vi "New Experiment.vi"(3 "error in (no error)":errorcluster, 4 "Experiment in":T1, 5 "Database.lvlib:Data Store.lvclass":refnum<class "Data Store.lvclass">) -> (0 "error out":errorcluster, 1 "Experiment out":T1, 2 "Database.lvlib:Data Store.lvclass 2":refnum<class "Data Store.lvclass">)   [LabVIEW 2012, in "Database.lvlib" / "Data Store.lvclass"]
uses:
  Data Store.lvclass
  Experiment.ctl
  <vilib>/addons/database/Auxilliary.llb/DB Tools Isolation Level.ctl
  <vilib>/addons/database/Auxilliary.llb/DB Tools Transaction.ctl
  Data Store.lvclass/Data Store.ctl
  <vilib>/addons/database/Connection.llb/Conn Transaction.vi
  <vilib>/addons/database/Connection.llb/Conn Execute.vi
  <vilib>/addons/database/Recordset.llb/Rec Fetch Integer Data (R).vi
  <vilib>/addons/database/Recordset.llb/Rec Destroy - Connection.vi
  <vilib>/addons/database/NI_Database_API.lvlib
  Database.lvlib
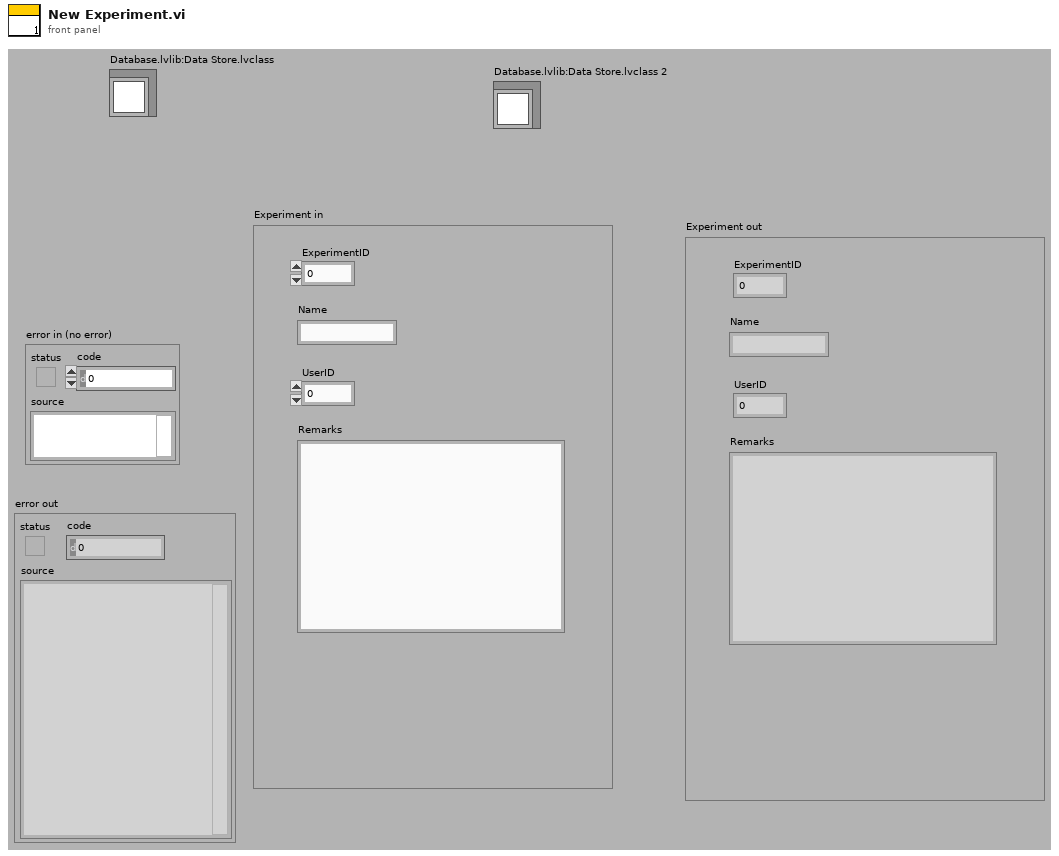
[diagram p1: front panel]
types:
  T1 = typedef "Database.lvlib/Experiment.ctl" = cluster{"ExperimentID":i32, "Name":string, "UserID":i32, "Remarks":string}
  T2 = typedef "NI_Database_API.lvlib/DB Tools Transaction.ctl" = enum16{"begin", "commit", "rollback"}
  T3 = typedef "NI_Database_API.lvlib/DB Tools Isolation Level.ctl" = enum16{"chaos", "read uncommitted", "read committed", "repeatable read", "serializable"}
  T4 = typedef "NI_Database_API.lvlib/Conn ObjectReference.ctl" = refnum<k1>
  T5 = typedef "NI_Database_API.lvlib/Rec ObjectReference.ctl" = refnum<k1>
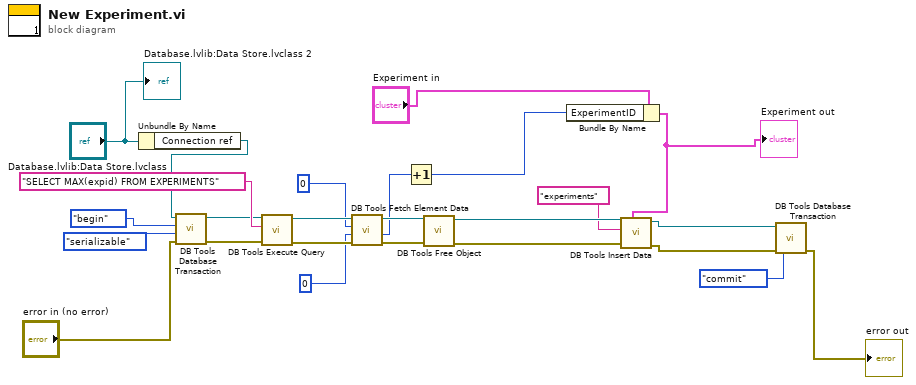
[diagram p0: block diagram]
diagram:
  n1 = Unbundle By Name("Database.lvlib:Data Store.lvclass") -> ("Connection ref"=w22:T4)
  n2 = call-poly <vilib>:"DB Tools Database Transaction.vi"("error in (no error)"="error in (no error)", "isolation level (chaos)"=DB_Tools_Isolation_Level."serializable", "operation (begin)"=DB_Tools_Transaction."begin", "connection reference"=w22) -> ("error out"=w18:errorcluster, "connection reference out"=w19:T4)  [unwired: 2 in]
  n3 = call-poly <vilib>:"DB Tools Execute Query.vi"("error in (no error)"=w18, "SQL query"="SELECT MAX(expid) FROM EXPERIMENTS", "connection reference"=w19) -> ("error out"=w16:errorcluster, "recordset reference"=w17:T5)  [unwired: 5 in]
  n4 = call-poly <vilib>:"DB Tools Fetch Element Data.vi"("error in (no error)"=w16, "type"=0, "column index"=0, "recordset reference"=w17) -> ("error out"=w13:errorcluster, "data"=w9:i32, "recordset reference out"=w12:T5)  [unwired: 3 in]
  n5 = Increment(x=w9) -> (x+1=w3:i32)
  n6 = call-poly <vilib>:"DB Tools Free Object.vi"("error in (no error)"=w13, "recordset reference"=w12) -> ("error out"=w8:errorcluster, "connection reference"=w7:T4)  [unwired: 8 in]
  n7 = Bundle By Name(cluster="Experiment in", "ExperimentID"=w3) -> (w1:T1)
  "Experiment out" <- w1
  n8 = call <vilib>:"DB Tools Insert Data.vi"("data"=w1, "error in (no error)"=w8, "table"="experiments", "connection reference"=w7) -> ("error out"=w4:errorcluster, "connection reference out"=w5:T4)  [unwired: 6 in]
  n9 = call-poly <vilib>:"DB Tools Database Transaction.vi"("error in (no error)"=w4, "operation (begin)"=DB_Tools_Transaction."commit", "connection reference"=w5) -> ("error out"=→"error out":errorcluster)  [unwired: 3 in, 1 out]
  "Database.lvlib:Data Store.lvclass 2" <- "Database.lvlib:Data Store.lvclass"
